vi "StoreClassesPaths.vi"(8 "error in":errorcluster, 10 "start path":path, 11 "CEF_Repository in":refnum<class "CEF_Repository.lvclass">) -> (0 "error out":errorcluster, 3 "CEF_Repository out":refnum<class "CEF_Repository.lvclass">)   [LabVIEW 2023, in "CEF.lvlib" / "CEF_Repository.lvclass"]
doc: "Stores the paths and classes name that the repo use.\n The default behavior is to store the path to the main folder containing the classes. If a more complex file structure is required this file needs to find all the classes and store the name and path pairs.\nCopyright 2017 National Instruments Corporation\n\nLicensed under the Apache License, Version 2.0 (the \"License\"); you may not use this file except in compliance with the License. You may obtain a copy of the License at http://www.apache.org/licenses/LICENSE-2.0\nUnless required by applicable law or agreed to in writing, software distributed under the License is distributed on an \"AS IS\" BASIS, WITHOUT WARRANTIES OR CONDITIONS OF ANY KIND, either express or implied. See the License for the specific language governing permissions and limitations under the License."
uses:
  CEF_Repository.lvclass
  class discovery singleton/class discovery singleton methods.ctl
  CEF.lvlib
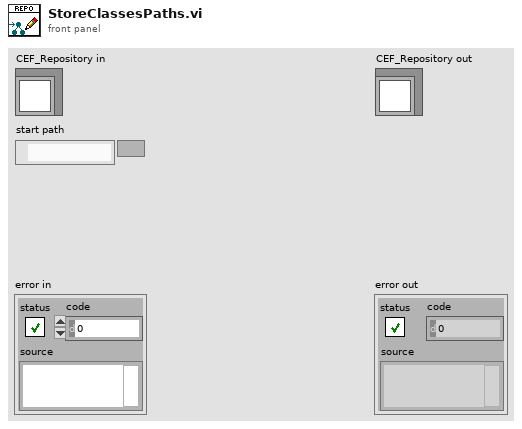
[diagram p1: front panel]
types:
  T1 = typedef "CEF.lvlib/class discovery singleton methods.ctl" = enum16{"add search paths", "load class by name", "list available classes", "get class path", "delete cache"}
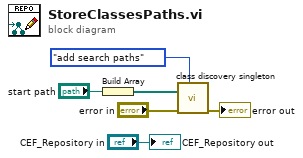
[diagram p0: block diagram]
diagram:
  n1 = Build Array("start path") -> (w1:path[])
  n2 = call "class discovery singleton.vi"("method"=class_discovery_singleton_methods."add search paths", "error in"="error in", "Plugin Search Paths"=w1) -> ("error out"=→"error out":errorcluster)  [unwired: 5 in, 3 out]
  "CEF_Repository out" <- "CEF_Repository in"
